vi "Read Waveform.vi"   [LabVIEW 2015, in "ZhiYuan ZDS Series for TCP.lvlib"]
doc: "Allows users to read one or more waveforms from the oscilloscope."
uses:
  ZhiYuan ZDS Series for TCP.lvlib
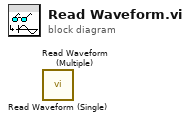
[diagram p0: block diagram]
diagram:
  n1 = call "Read Waveform (Single).vi"() -> ()  [unwired: 9 in, 3 out]
  n2 = call "Read Waveform (Multiple).vi"() -> ()  [unwired: 9 in, 3 out]
